vi "setTaskRef.vi"(8 "error in (no error)":errorcluster, 10 "DAQmx Task Ref":refnum<k21>, 11 "niDAQmxAO.lvclass in":refnum<class "niDAQmxAO.lvclass">) -> (0 "error out":errorcluster, 3 "niDAQmxAO.lvclass out":refnum<class "niDAQmxAO.lvclass">)   [LabVIEW 2011, in "Hardware.lvlib" / "Channels.lvlib" / "niDAQmxAO.lvclass"]
uses:
  niDAQmxAO.lvclass
  niDAQmxAO.lvclass/niDAQmxAO.ctl
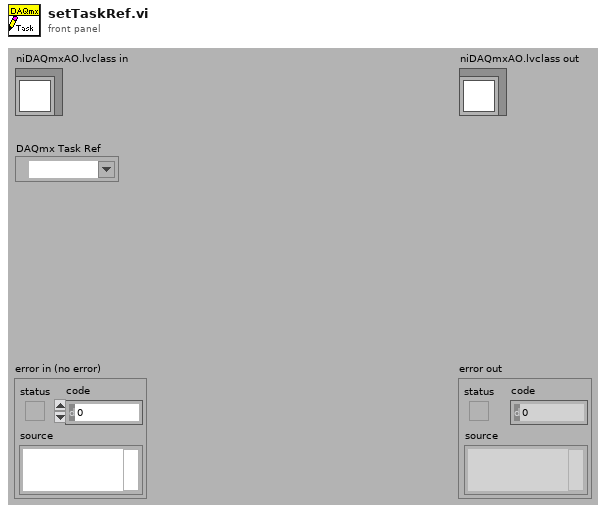
[diagram p1: front panel]
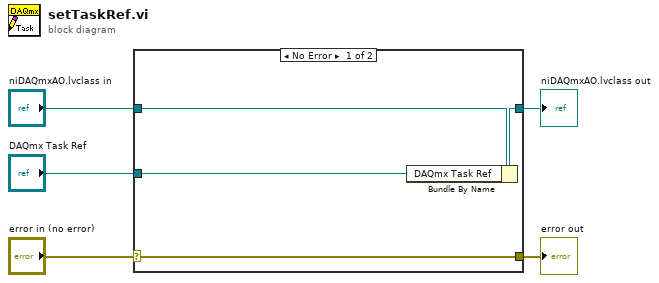
[diagram p0: block diagram]
diagram:
  n1 = case shown="No Error" "error in (no error)" {
    selector: "error in (no error)" -> [w9 w10]
    tunnel: [w9 w10] -> w4
    tunnel: [w7 w11] -> w2
    tunnel: "niDAQmxAO.lvclass in" -> [w8 w11]
    tunnel: "DAQmx Task Ref" -> [w6 _]
    frame No Error {
      n2 = Bundle By Name(cluster=w8, "DAQmx Task Ref"=w6) -> (w7:refnum<class "niDAQmxAO.lvclass">)
    }
    frame Error {
    }
  }
  "error out" <- w4
  "niDAQmxAO.lvclass out" <- w2
